vi "右相机穿管检测CCD2.vi"(8 "error in (no error)":errorcluster caption="错误输入（无错误）", 11 "名称或相对路径":string="Template Program") -> (0 "error in (no error) 2":errorcluster caption="错误输入（无错误）")   [LabVIEW 2017]
uses:
  Picture/SaveButtom.ctl
  <vilib>/vision/Pattern Matching.llb/IMAQ Curve Parameters.ctl
  Global System.vi
  <vilib>/Utility/xml.llb/Write to XML File(string).vi
panel:
  in  "ROI BIG 获取":bool
  in  "获取图像":bool
  in  "ROI LINE 获取":bool
  in  "创建模板":bool
  in  "保存图像":bool
  out "添加的路径":path
  in  "刷新":bool
  in  "测试按钮":bool
  in  "保存按钮":bool
  in  "Main":enum32{"主参数", "模板匹配参数 ", "CCD2 ROI参数", "测试效果"}(tab)
  in  "CCD2基础参数":T1={"IsNorImage"=TRUE, "Exposure Values"=100289, "ImagePath"=path "C:/Users/hedongpo/Desktop/514-hdp/Alignment Assemble System/Test Picture/B/3.bmp"} caption="参数界面" {"Exposure Values" scale=0.0..200000.0}
  in  "CCD2参数":T4={"Rectangle"={"Left"=1952, "Top"=146, "Right"=370, "Bottom"=2690, "Rotation"=45.0}, "Angle (degrees) "=90.0, "long"=150.0, "abgek"=-90.0, "Color"=16711680, "left threshold"=0.0, "Rectangle right"={"Left"=1952, "Top"=1596, "Right"=570, "Bottom"=2690, "Rotation"=45.0}, "long right"=150.0, "abgek right"=90.0, "Color 2"=16711680, "right threshold"=0.0, "left"=0.0, "right"=0.0, "Settings (Big)"={"Extraction Mode"=0, "Edge Threshold"=17, "Edge Filter Size"=1, "Min Length"=36, "Row Search Step Size"=13, "Col Search Step Size"=13, "Max Endpoint Gap"=10, "Closed"=FALSE, "Subpixel"=TRUE}, "Clamp Settings (Big)"={"Angle "=10.0, "Edge Polarity"={"Start"=0, "End"=0}}, " Settings top"={"Extraction Mode"=0, "Edge Threshold"=18, "Edge Filter Size"=1, "Min Length"=36, "Row Search Step Size"=64, "Col Search Step Size"=64, "Max Endpoint Gap"=10, "Closed"=FALSE, "Subpixel"=TRUE}, "Clamp Settings top "={"Angle "=10.0, "Edge Polarity"={"Start"=0, "End"=0}}, "Sub-Pixel Accuracy "=TRUE, "Threshold Parameters"={"Level Type"=enum."Absolute Value", "Threshold Level"=127, "Hysteresis"=2}, "Process "=enum."Get First + Last Edge", "Threshold Parameters 2"={"Level Type"=enum."Absolute Value", "Threshold Level"=127, "Hysteresis"=2}} {"Clamp Settings top"."Edge Polarity"."Start" items=["Any", "Rising", "Falling"]; "Clamp Settings top"."Edge Polarity"."End" items=["Any", "Rising", "Falling"]; "Settings top"."Extraction Mode" items=["Normal", "Uniform Regions"]; "Settings top"."Edge Filter Size" items=["Fine", "Normal", "Contour Tracing"]; "Settings top"."Max Endpoint Gap" min=0; "Settings top"."Col Search Step Size" min=1 max=255 step=1; "Settings top"."Row Search Step Size" min=1 max=255 step=1; "Settings top"."Min Length" min=0; "Settings top"."Edge Threshold" min=1 max=350 step=1; "Clamp Settings (Big)"."Edge Polarity"."Start" items=["Any", "Rising", "Falling"]; "Clamp Settings (Big)"."Edge Polarity"."End" items=["Any", "Rising", "Falling"]; "Settings (Big)"."Extraction Mode" items=["Normal", "Uniform Regions"]; "Settings (Big)"."Edge Filter Size" items=["Fine", "Normal", "Contour Tracing"]; "Settings (Big)"."Max Endpoint Gap" min=0; "Settings (Big)"."Col Search Step Size" min=1 max=255 step=1; "Settings (Big)"."Row Search Step Size" min=1 max=255 step=1; "Settings (Big)"."Min Length" min=0; "Settings (Big)"."Edge Threshold" min=1 max=350 step=1; "Rectangle right"."Rotation" format="%.2f"; "Rectangle right"."Left" scale=0.0..1024.0; "Rectangle right"."Right" scale=0.0..1024.0; "Rectangle"."Rotation" format="%.2f"; "Rectangle"."Left" scale=0.0..1024.0; "Rectangle"."Right" scale=0.0..1024.0}
  in  "CCD2 ROI参数":T6={"Rectangle big CCD1"={"Left"=1952, "Top"=1596, "Right"=570, "Bottom"=2690, "Rotation"=45.0}, "Rectangle top CCD1 "={"Left"=1952, "Top"=1596, "Right"=570, "Bottom"=2690, "Rotation"=45.0}, "Line"={"Start X"=0, "Start Y"=0, "End X"=0, "End Y"=0}, "left line "=846.0, "right line"=1152.0} {"Line"."Start X" scale=0.0..1024.0; "Line"."End X" scale=0.0..1024.0; "Rectangle top CCD1"."Rotation" format="%.2f"; "Rectangle top CCD1"."Left" scale=0.0..1024.0; "Rectangle top CCD1"."Right" scale=0.0..1024.0; "Rectangle big CCD1"."Rotation" format="%.2f"; "Rectangle big CCD1"."Left" scale=0.0..1024.0; "Rectangle big CCD1"."Right" scale=0.0..1024.0}
  out "原始图像":T7(plugin-control)
  out "路径输出":path
  in  "Vision Paramter Save Buttom":T8
  out "system time":string
  in  "确认按钮":bool
  # "箭头指示参数"
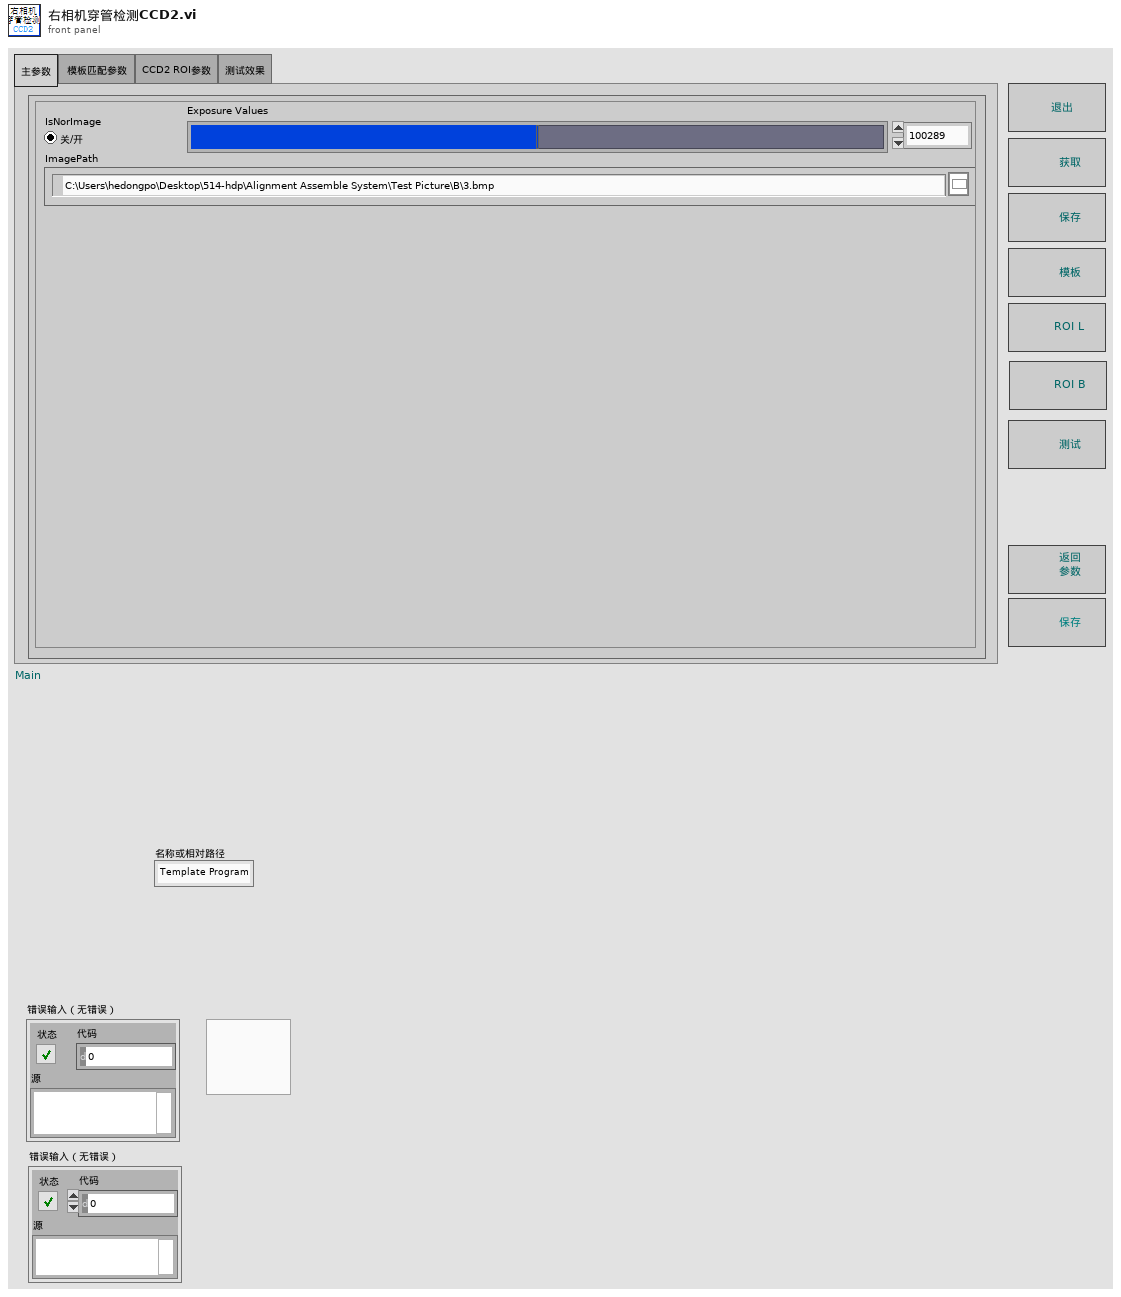
[diagram p1: front panel]
types:
  T1 = cluster{"IsNorImage":bool, "Exposure Values":u32, "ImagePath":path}
  T2 = typedef "IMAQ Rectangle" = cluster{"Left":i32, "Top":i32, "Right":i32, "Bottom":i32, "Rotation":dbl}
  T3 = typedef "IMAQ Curve Parameters.ctl" = cluster{"Extraction Mode":u32, "Edge Threshold":i32, "Edge Filter Size":u32, "Min Length":i32, "Row Search Step Size":i32, "Col Search Step Size":i32, "Max Endpoint Gap":i32, "Closed":bool, "Subpixel":bool}
  T4 = cluster{"Rectangle":T2, "Angle (degrees) ":sgl, "long":sgl, "abgek":dbl, "Color":u32, "left threshold":dbl, "Rectangle right":T2, "long right":sgl, "abgek right":dbl, "Color 2":u32, "right threshold":dbl, "left":dbl, "right":dbl, "Settings (Big)":T3, "Clamp Settings (Big)":cluster{"Angle ":dbl, "Edge Polarity":cluster{"Start":u32, "End":u32}}, " Settings top":T3, "Clamp Settings top ":cluster{"Angle ":dbl, "Edge Polarity":cluster{"Start":u32, "End":u32}}, "Sub-Pixel Accuracy ":bool, "Threshold Parameters":cluster{"Level Type":enum32{"Absolute Value", "Relative value"}, "Threshold Level":i32, "Hysteresis":i32}, "Process ":enum16{"Get First Edge", "Get First + Last Edge", "Get All Edges"}, "Threshold Parameters 2":cluster{"Level Type":enum32{"Absolute Value", "Relative value"}, "Threshold Level":i32, "Hysteresis":i32}}
  T5 = typedef "IMAQ Line" = cluster{"Start X":i32, "Start Y":i32, "End X":i32, "End Y":i32}
  T6 = cluster{"Rectangle big CCD1":T2, "Rectangle top CCD1 ":T2, "Line":T5, "left line ":dbl, "right line":dbl}
  T7 = typedef "IMAQ Image.ctl" = refnum<image>
  T8 = typedef "SaveButtom.ctl" = bool
  T9 = cluster{"index":i32, "this vi":refnum<vi>, "error out":errorcluster}
  T10 = cluster{"master data":string, "priority":u16, "secondary data":string[]}
  T11 = cluster{"case name":string[], "queue array":refnum<queue>[]}
  T12 = typedef "IMAQdx.ctl" = refnum<k21>
  T13 = cluster{"Global Rectangle":i32[], "Contours":cluster{"Contour Type":u32, "ROI Type":u32, "Points":i32[]}[]}
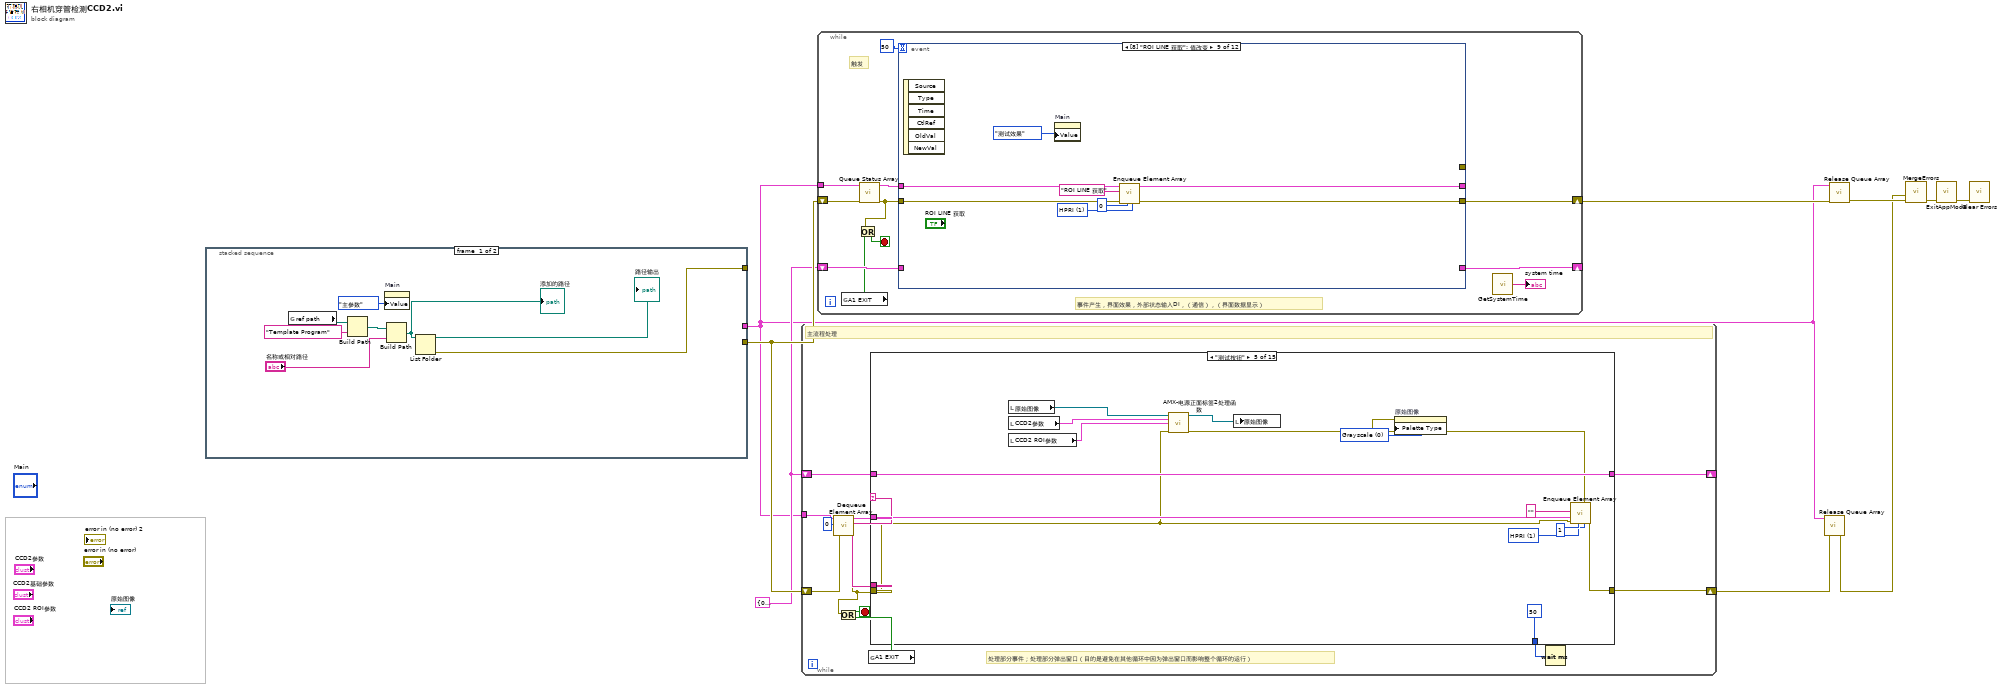
[diagram p0: block diagram]
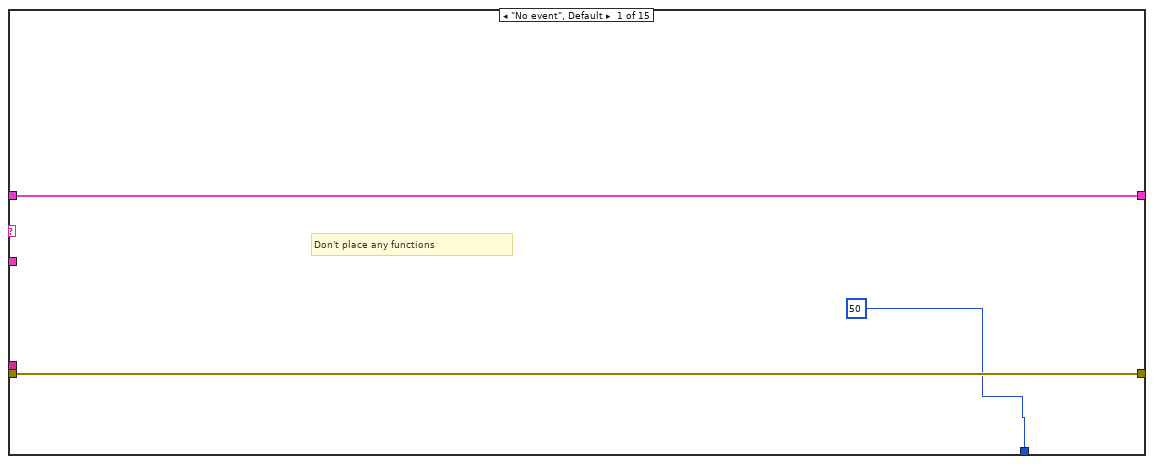
[diagram p2: hidden frame]
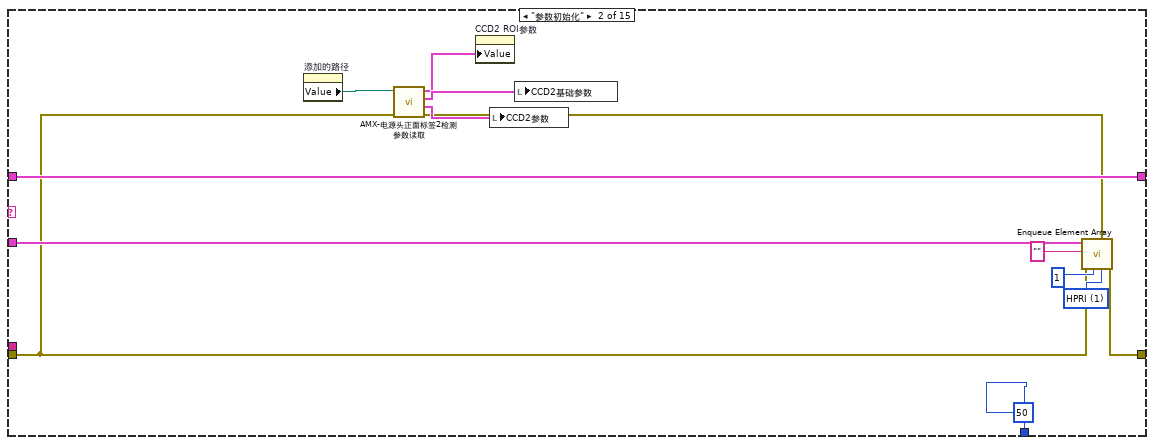
[diagram p3: hidden frame]
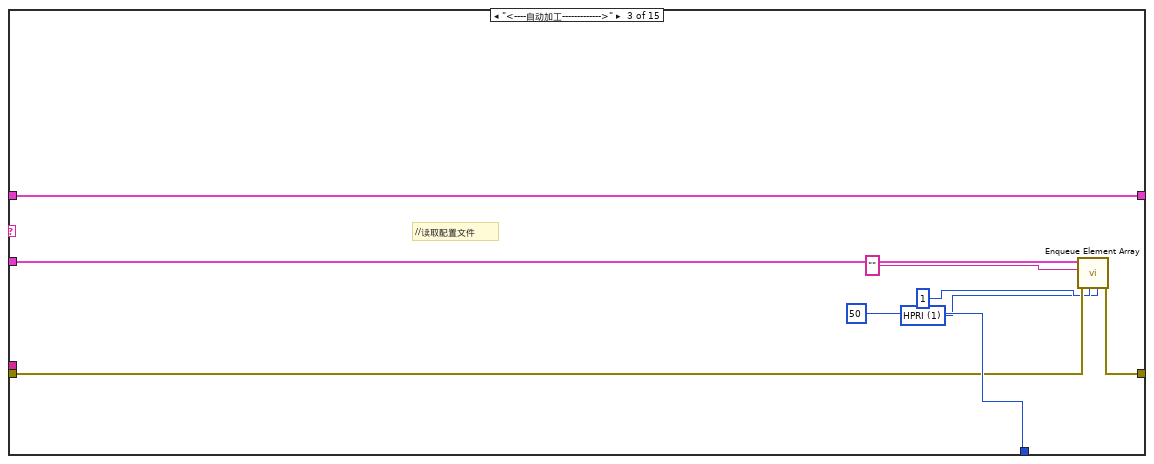
[diagram p4: hidden frame]
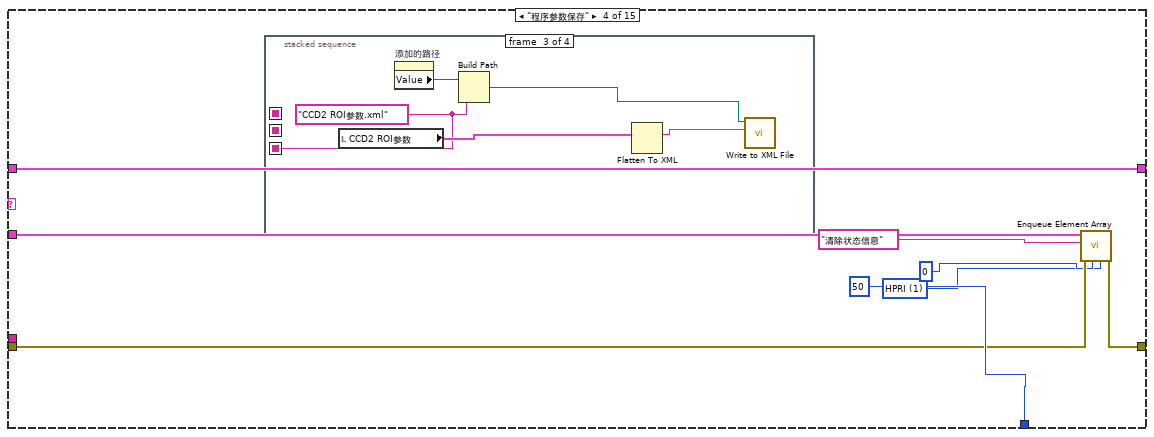
[diagram p5: hidden frame]
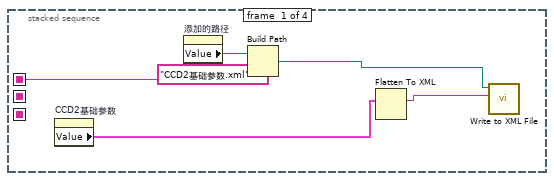
[diagram p6: hidden frame]
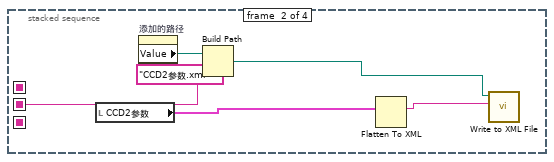
[diagram p7: hidden frame]
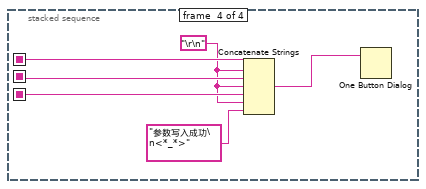
[diagram p8: hidden frame]
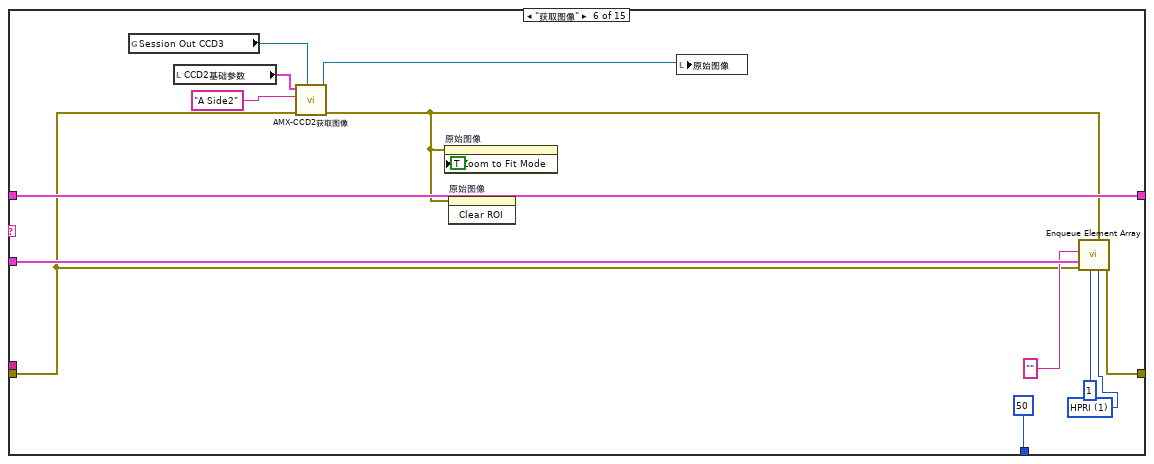
[diagram p9: hidden frame]
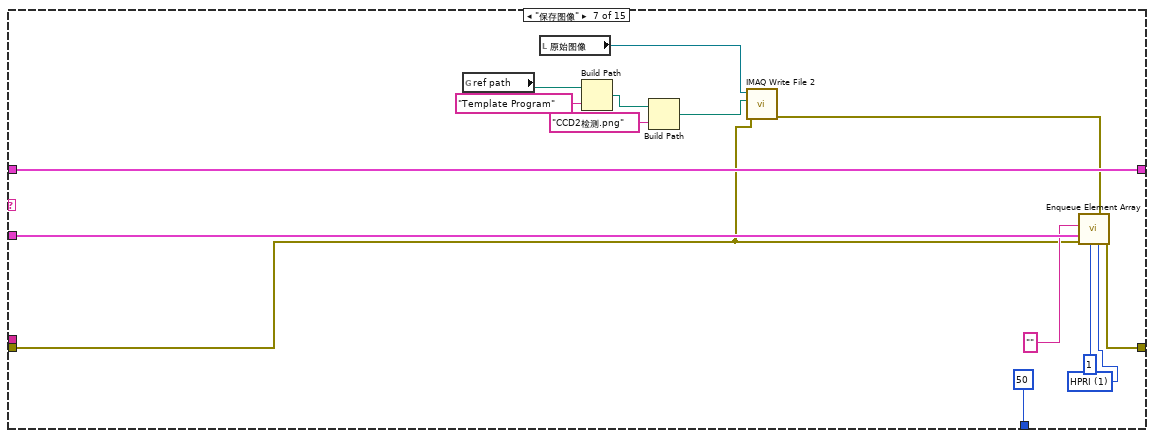
[diagram p10: hidden frame]
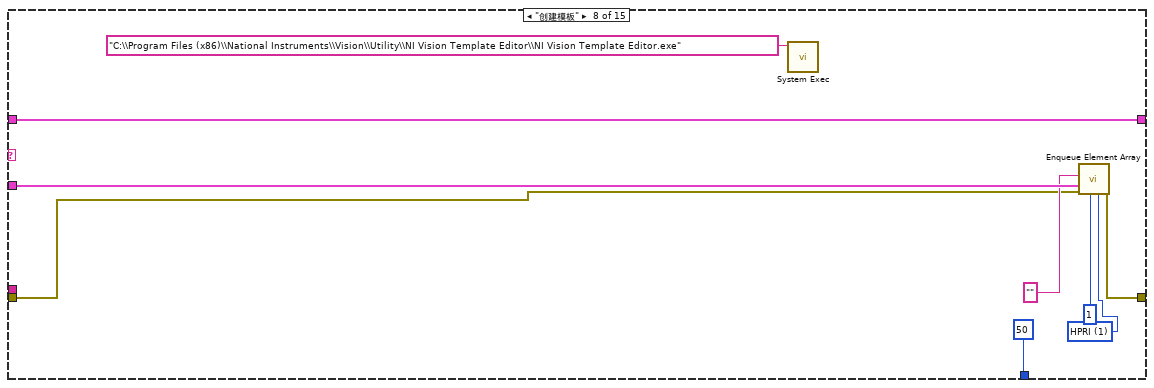
[diagram p11: hidden frame]
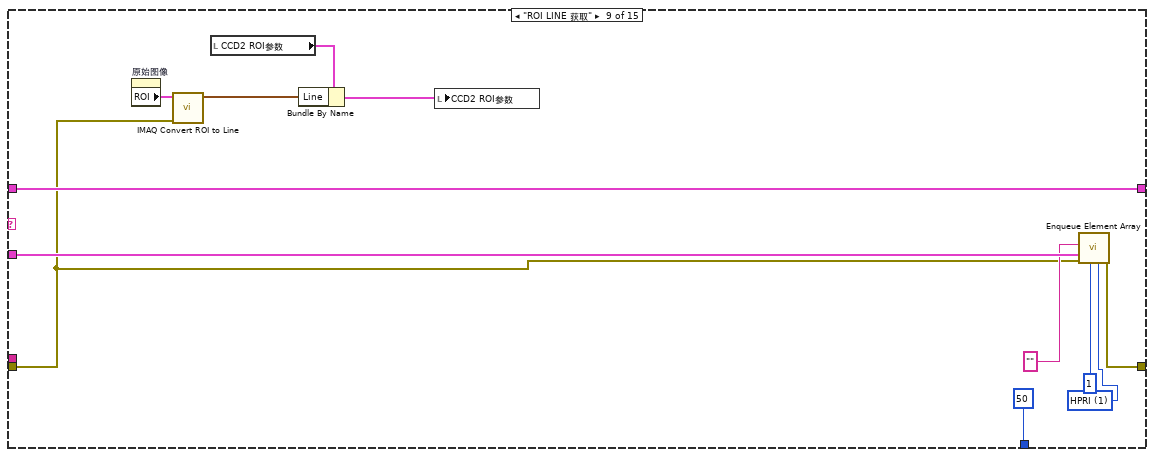
[diagram p12: hidden frame]
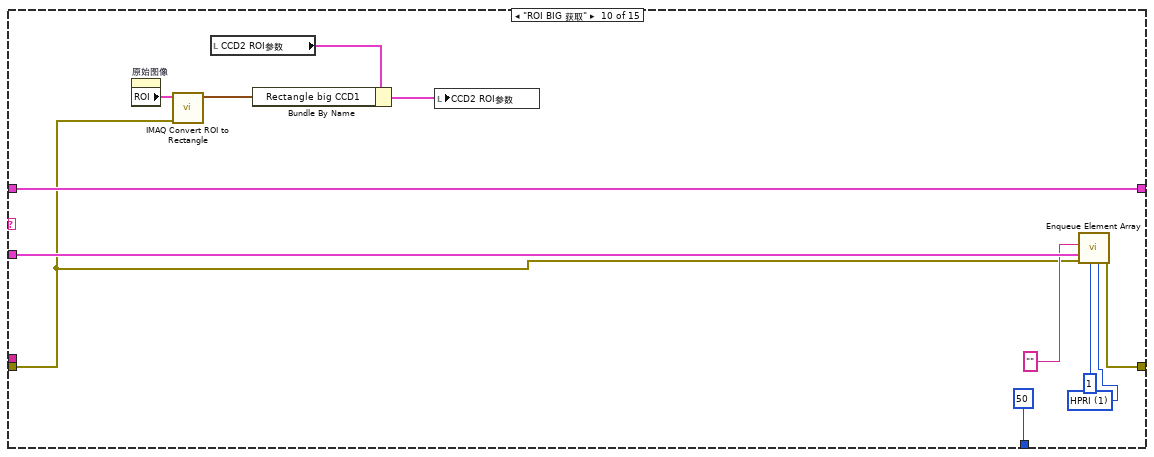
[diagram p13: hidden frame]
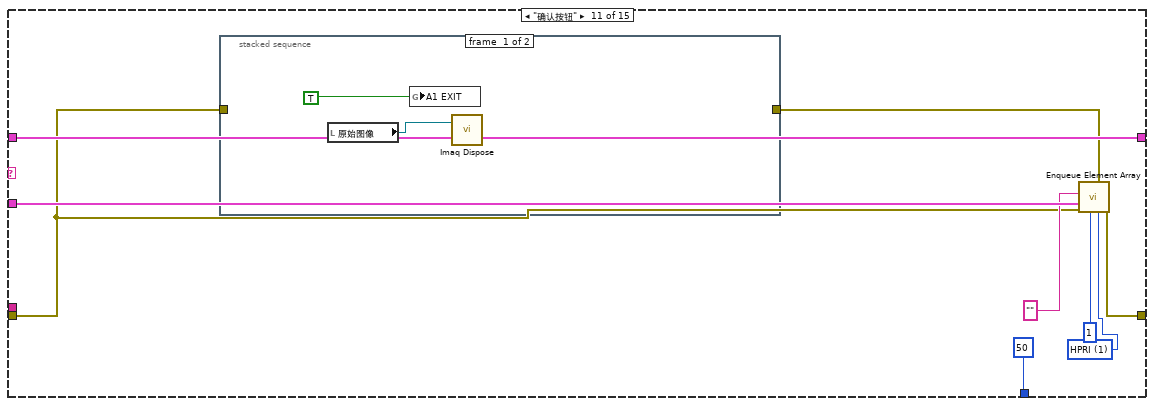
[diagram p14: hidden frame]
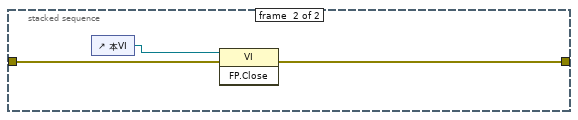
[diagram p15: hidden frame]
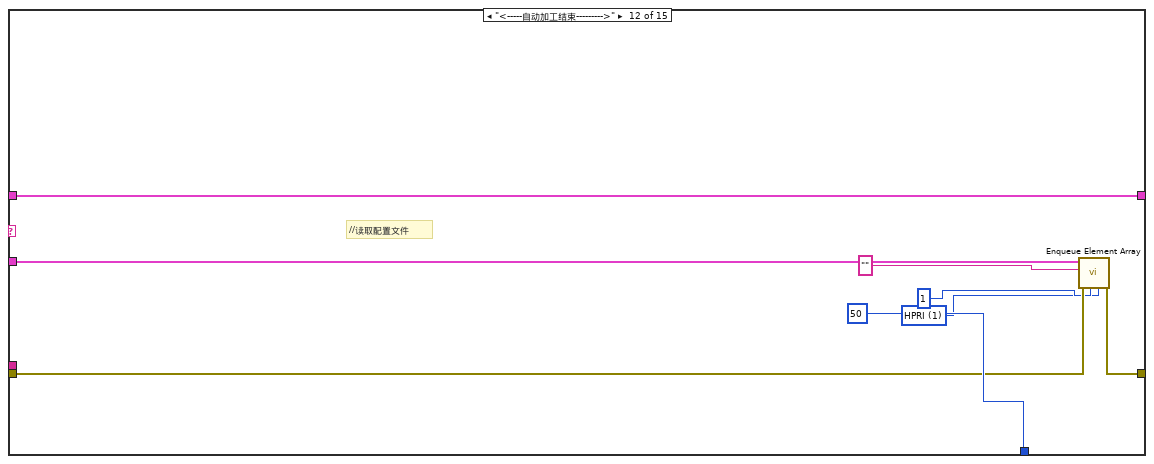
[diagram p16: hidden frame]
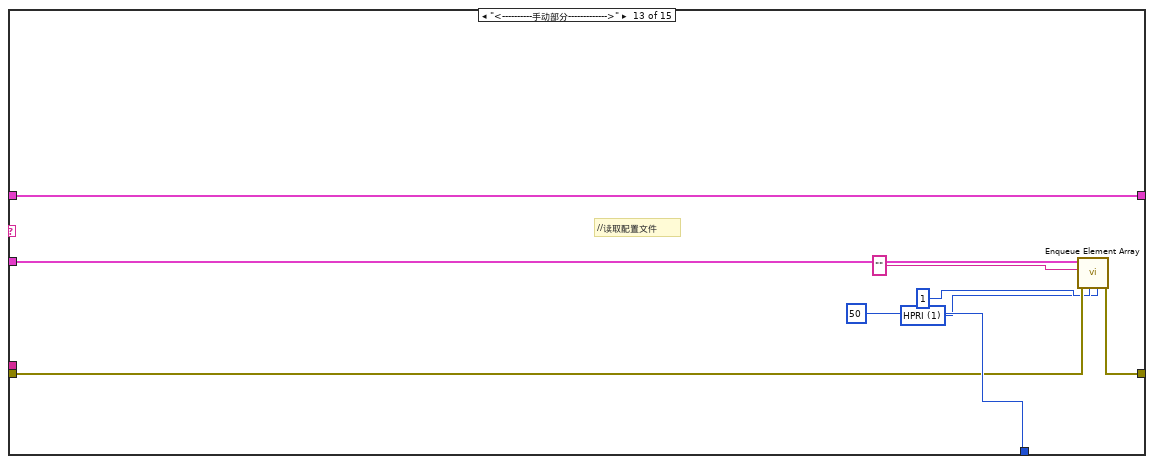
[diagram p17: hidden frame]
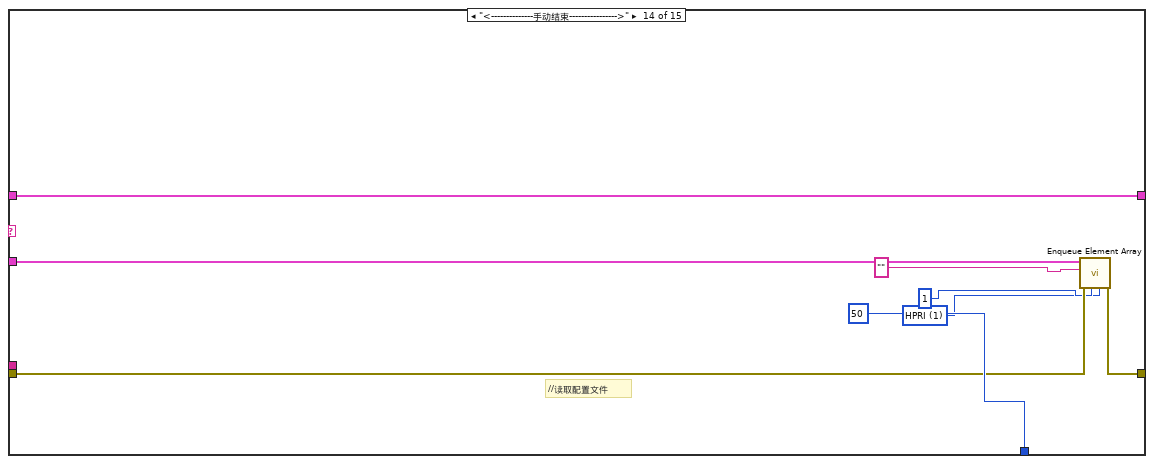
[diagram p18: hidden frame]
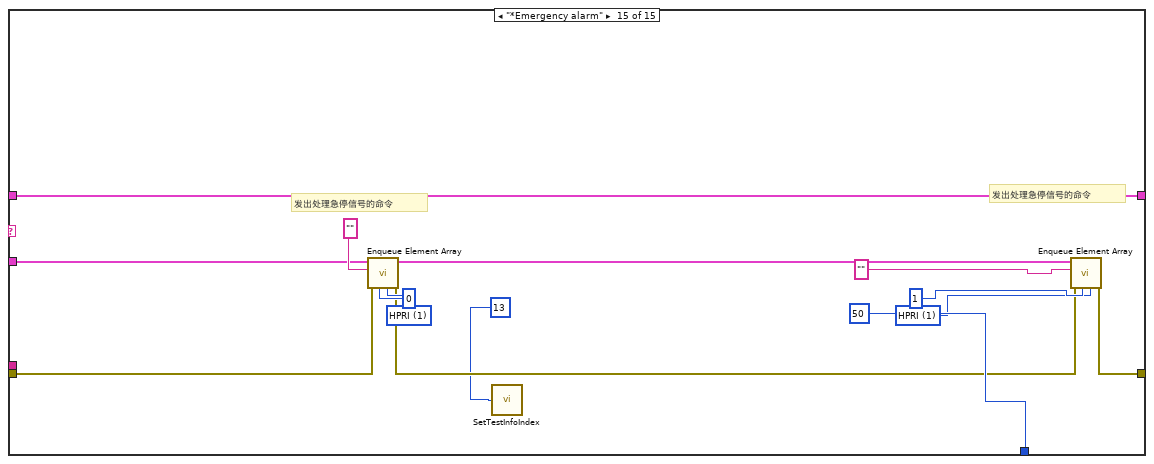
[diagram p19: hidden frame]
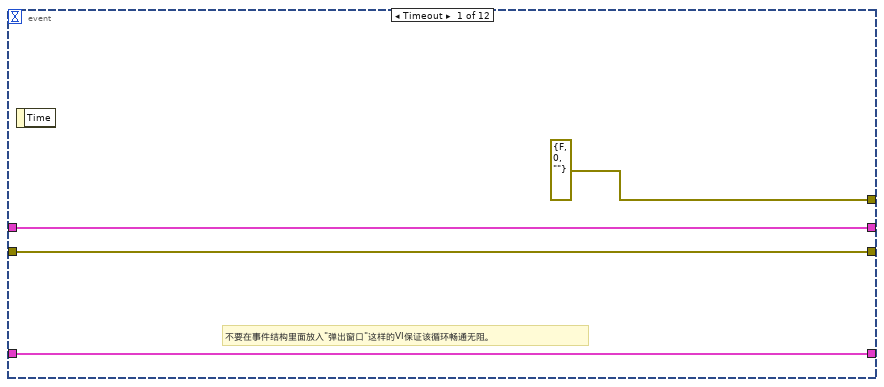
[diagram p20: hidden frame]
diagram:
  w4 = T9 {"index"=0, "this vi"=refnum, "error out"={"status"=FALSE, "code"=0, "source"=""}} ("parameter buffer")
  n1 = stacked-sequence {
    tunnel: [w15 _] -> _
    tunnel: [_ w19] -> w5
    tunnel: [_ w18] -> w1
    frame #0 {
      n2 = global read "Global System.vi" "ref path"() -> (w13:path)
      n3 = Build Path(base path=w13, name or relative path="Template Program" ("名称或相对路径")) -> (appended path=w11:path)
      n4 = property on="Main" class="TabCtl (严格)"("Value"=enum32{"主参数", "模板匹配参数 ", "CCD2 ROI参数", "测试效果"}."主参数" ("Main")) -> ()  [unwired: 2 in, 2 out]
      n5 = Build Path(base path=w11, name or relative path="名称或相对路径") -> (appended path=w17:path)
      "添加的路径" <- w17
      n6 = List Folder(path=w17) -> (path out=→"路径输出":path, error out=w15:errorcluster)  [unwired: 3 in, 2 out]
    }
    frame #1 {
      w27 = string[] ["comm queue1", "data queue 11", "data queue 12", "data queue 13", "data queue 14"]  # queue name
      w28 = 4  # queue num
      w29 = T10 {"master data"="", "priority"=0, "secondary data"=[]}  # element data type
      n7 = call "Obtain Queue Array.vi"("queue name"=w27, "element data type"=w29, "queue num"=w28) -> ("error out"=w23:errorcluster, "queue out"=w24:T11)  [unwired: 2 in, 1 out]
      n8 = call "Enqueue Element Array.vi"("queue index"=0, "error in"=w23, "master data"="参数初始化", "queue in"=w24) -> ("error out"=w22:errorcluster, "queue out"=w21:T11)  [unwired: 6 in]
      n9 = disable-structure shown="启用" {
        disable-tunnel: w22 -> [w35 w36]
        disable-tunnel: w21 -> [w34 w37]
        disable-tunnel: "Loading Variable" ("master data") -> [w33 _]
        disable-tunnel: [w31 w36] -> w19
        disable-tunnel: [w30 w37] -> w18
        frame Disabled {
          n10 = call "Enqueue Element Array.vi"("queue index"=12, "error in"=w35, "master data"=w33, "queue in"=w34) -> ("error out"=w31:errorcluster, "queue out"=w30:T11)  [unwired: 6 in]
        }
        frame Enabled {
        }
      }
    }
  }
  n11 = while {
    shift-right: [w50] -> w3
    shift-left: w5 -> [w41]
    shift-right: [w47] -> _
    shift-left: w4 -> [w48]
    tunnel: w1 -> [w43]
    stop <- w38 stop-if-true
    # "处理部分事件；处理部分弹出窗口（目的是避免在其他循环中因为弹出窗口而影响整个循环的运行）"
    # "主流程处理"
    n12 = call "Dequeue Element Array.vi"("queue in"=w43, "queue index"=0, "error in"=w41) -> ("queue out"=w46:T11, "master data"=w45:string, "secondary data"=w44:string[], "error out"=w40:errorcluster)  [unwired: 2 in, 1 out]
    n13 = global read "Global System.vi" "A1 EXIT"() -> (w39:bool)
    n14 = Or(x=w40, y=w39) -> (x .or. y?=w38:bool)
    n15 = case shown="\"测试按钮\"" w45 {
      tunnel: w46 -> [_ w65 w73 w75 w116 w130 w145 w154 w166 w178 w187 w200 w208 w216 w222]
      tunnel: w40 -> [w52 w58 w69 w79 w110 w121 w132 w148 w159 w171 w181 w196 w204 w212 w219]
      tunnel: [w52 w64 w72 w81 w115 w129 w144 w153 w165 w177 w186 w199 w207 w215 w230] -> w50
      tunnel: [50 50 50 50 50 50 50 50 50 50 50 50 50 50 50] -> w49
      tunnel: w48 -> [w53 w60 w70 w76 w111 w125 w140 w149 w161 w173 w182 w197 w205 w213 w228]
      tunnel: [w53 w60 w70 w76 w111 w125 w140 w149 w161 w173 w182 w197 w205 w213 w228] -> w47
      tunnel: w44 -> [_ _ _ _ _ _ _ _ _ _ _ _ _ _ _]
      frame "No event", Default {
        # "Don't place any functions"
      }
      frame "参数初始化" {
        w61 = u16 1 items=["HPRI"=1, "LPRI"=0] ("priority")
        n16 = property on="添加的路径" class="Path"() -> ("Value"=w59:path)  [unwired: 2 in, 2 out]
        n17 = call "AMX-电源头正面标签2检测参数读取.vi"("error in (no error)"=w58, "基路径"=w59) -> ("error out"=w55:errorcluster, "CCD2参数"=w56:T4, "CCD2基础参数"=w57:T1, "CCD2 ROI参数"=w54:T6)  [unwired: 5 in]
        n18 = property on="CCD2 ROI参数" class="Clust (严格)"("Value"=w54) -> ()  [unwired: 2 in, 2 out]
        n19 = local write "CCD2参数"(w56) -> ()
        n20 = local write "CCD2基础参数"(w57) -> ()
        n21 = call "Enqueue Element Array.vi"("priority"=w61, "device error in"=w55, "queue index"=1, "error in"=w58, "master data"="" ("Element 1"), "queue in"=w65) -> ("error out"=w64:errorcluster)  [unwired: 4 in, 1 out]
      }
      frame "<----自动加工------------->" {
        w67 = u16 1 items=["HPRI"=1, "LPRI"=0] ("priority")
        # "//读取配置文件"
        n22 = call "Enqueue Element Array.vi"("priority"=w67, "queue index"=1, "error in"=w69, "master data"="" ("Element 1"), "queue in"=w73) -> ("error out"=w72:errorcluster)  [unwired: 5 in, 1 out]
      }
      frame "程序参数保存" {
        w77 = u16 1 items=["HPRI"=1, "LPRI"=0] ("priority")
        n23 = stacked-sequence {
          seq-local: [w83 _ _ _] -> [_ _ _ w103]
          seq-local: [_ w89 _ _] -> [_ _ _ w101]
          seq-local: [_ _ w93 _] -> [_ _ _ w99]
          frame #0 {
            w83 = "CCD2基础参数.xml" ("名称或相对路径")
            n24 = property on="CCD2基础参数" class="Clust (严格)"() -> ("Value"=w86:T1)  [unwired: 2 in, 2 out]
            n25 = property on="添加的路径" class="Path"() -> ("Value"=w87:path)  [unwired: 2 in, 2 out]
            n26 = Build Path(base path=w87, name or relative path=w83) -> (appended path=w84:path)
            n27 = Flatten To XML(anything=w86) -> (xml string=w85:string)
            n28 = call-poly <vilib>:"Write to XML File.vi"("XML Input"=w85, "XML File Path"=w84) -> ()  [unwired: 7 in, 3 out]
          }
          frame #1 {
            w89 = "CCD2参数.xml" ("名称或相对路径")
            n29 = local read "CCD2参数"() -> (w88:T4)
            n30 = property on="添加的路径" class="Path"() -> ("Value"=w92:path)  [unwired: 2 in, 2 out]
            n31 = Build Path(base path=w92, name or relative path=w89) -> (appended path=w90:path)
            n32 = Flatten To XML(anything=w88) -> (xml string=w91:string)
            n33 = call-poly <vilib>:"Write to XML File.vi"("XML Input"=w91, "XML File Path"=w90) -> ()  [unwired: 7 in, 3 out]
          }
          frame #2 {
            w93 = "CCD2 ROI参数.xml" ("名称或相对路径")
            n34 = local read "CCD2 ROI参数"() -> (w94:T6)
            n35 = property on="添加的路径" class="Path"() -> ("Value"=w97:path)  [unwired: 2 in, 2 out]
            n36 = Build Path(base path=w97, name or relative path=w93) -> (appended path=w95:path)
            n37 = Flatten To XML(anything=w94) -> (xml string=w96:string)
            n38 = call-poly <vilib>:"Write to XML File.vi"("XML Input"=w96, "XML File Path"=w95) -> ()  [unwired: 7 in, 3 out]
          }
          frame #3 {
            w98 = "\r\n"
            n39 = Concatenate Strings(w103, w98, w101, w98, w99, w98, "参数写入成功\n<*_*>" ("消息")) -> (w102:string)
            n40 = One Button Dialog(message=w102) -> ()  [unwired: 1 in, 1 out]
          }
        }
        n41 = call "Enqueue Element Array.vi"("priority"=w77, "queue index"=0, "error in"=w79, "master data"="清除状态信息" ("Element 1"), "queue in"=w75) -> ("error out"=w81:errorcluster)  [unwired: 5 in, 1 out]
      }
      frame "测试按钮" {
        w106 = u32 0 items=["Grayscale", "Binary", "Gradient", "Rainbow", "Temperature", "User Defined", "Binary 16 Bit", "Gradient 16 Bit", "Rainbow 16 Bit", "Temperature 16 Bit", "User Defined 16 Bit"] ("Palette:Palette Type")
        w112 = u16 1 items=["HPRI"=1, "LPRI"=0] ("priority")
        n42 = local read "原始图像"() -> (w108:T7)
        n43 = local read "CCD2参数"() -> (w105:T4)
        n44 = local read "CCD2 ROI参数"() -> (w104:T6)
        n45 = call "AMX-电源正面标签2处理函数.vi"("Image in"=w108, "CCD2参数"=w105, "CCD2 ROI参数"=w104, "error in (no error)"=w110) -> ("Image out"=w109:T7, "error out"=w107:errorcluster)  [unwired: 7 in, 3 out]
        n46 = local write "原始图像"(w109) -> ()
        n47 = property on="原始图像" class="ImageControl"(error in=w107, "Palette Type"=w106) -> ()  [unwired: 1 in, 2 out]
        n48 = call "Enqueue Element Array.vi"("priority"=w112, "device error in"=w107, "queue index"=1, "error in"=w110, "master data"="" ("Element 1"), "queue in"=w116) -> ("error out"=w115:errorcluster)  [unwired: 4 in, 1 out]
      }
      frame "获取图像" {
        w126 = u16 1 items=["HPRI"=1, "LPRI"=0] ("priority")
        n49 = global read "Global System.vi" "Session Out CCD3"() -> (w118:T12)
        n50 = local read "CCD2基础参数"() -> (w123:T1)
        n51 = call "AMX-CCD2获取图像.vi"("Session Out CCD3"=w118, "error in (no error)"=w121, "Image Name"="A Side2", "ParamsUI"=w123) -> ("error out"=w119:errorcluster, "Image out"=w122:T7)  [unwired: 4 in, 2 out]
        n52 = property on="原始图像" class="ImageControl"(error in=w119, "Zoom to Fit Mode"=TRUE) -> ()  [unwired: 1 in, 2 out]
        n53 = invoke on="原始图像" class="ImageControl" method="Clear ROI"(error in=w119) -> ()  [unwired: 2 in, 3 out]
        n54 = local write "原始图像"(w122) -> ()
        n55 = call "Enqueue Element Array.vi"("priority"=w126, "device error in"=w119, "queue index"=1, "error in"=w121, "master data"="" ("Element 1"), "queue in"=w130) -> ("error out"=w129:errorcluster)  [unwired: 4 in, 1 out]
      }
      frame "保存图像" {
        w141 = u16 1 items=["HPRI"=1, "LPRI"=0] ("priority")
        n56 = global read "Global System.vi" "ref path"() -> (w139:path)
        n57 = local read "原始图像"() -> (w133:T7)
        n58 = Build Path(base path=w139, name or relative path="Template Program" ("名称或相对路径")) -> (appended path=w137:path)
        n59 = Build Path(base path=w137, name or relative path="CCD2检测.png" ("名称或相对路径")) -> (appended path=w135:path)
        n60 = call-poly "IMAQ Write File 2"("error in (no error)"=w132, "File Path"=w135, "Image"=w133) -> ("error out"=w134:errorcluster)  [unwired: 7 in, 1 out]
        n61 = call "Enqueue Element Array.vi"("priority"=w141, "device error in"=w134, "queue index"=1, "error in"=w132, "master data"="" ("Element 1"), "queue in"=w145) -> ("error out"=w144:errorcluster)  [unwired: 4 in, 1 out]
      }
      frame "创建模板" {
        w150 = u16 1 items=["HPRI"=1, "LPRI"=0] ("priority")
        n62 = call <vilib>:"System Exec.vi"("command line"="C:\\Program Files (x86)\\National Instruments\\Vision\\Utility\\NI Vision Template Editor\\NI Vision Template Editor.exe") -> ()  [unwired: 7 in, 4 out]
        n63 = call "Enqueue Element Array.vi"("priority"=w150, "queue index"=1, "error in"=w148, "master data"="" ("Element 1"), "queue in"=w154) -> ("error out"=w153:errorcluster)  [unwired: 5 in, 1 out]
      }
      frame "ROI LINE 获取" {
        w162 = u16 1 items=["HPRI"=1, "LPRI"=0] ("priority")
        n64 = property on="原始图像" class="ImageControl"() -> ("ROI"=w160:T13)  [unwired: 2 in, 2 out]
        n65 = call "IMAQ Convert ROI to Line"("error in (no error)"=w159, "ROI Descriptor"=w160) -> ("Line"=w157:T5)  [unwired: 7 in, 1 out]
        n66 = local read "CCD2 ROI参数"() -> (w158:T6)
        n67 = Bundle By Name(cluster=w158, "Line"=w157) -> (w156:T6)
        n68 = local write "CCD2 ROI参数"(w156) -> ()
        n69 = call "Enqueue Element Array.vi"("priority"=w162, "queue index"=1, "error in"=w159, "master data"="" ("Element 1"), "queue in"=w166) -> ("error out"=w165:errorcluster)  [unwired: 5 in, 1 out]
      }
      frame "ROI BIG 获取" {
        w174 = u16 1 items=["HPRI"=1, "LPRI"=0] ("priority")
        n70 = property on="原始图像" class="ImageControl"() -> ("ROI"=w172:T13)  [unwired: 2 in, 2 out]
        n71 = call "IMAQ Convert ROI to Rectangle"("error in (no error)"=w171, "ROI Descriptor"=w172) -> ("Rectangle"=w169:T2)  [unwired: 7 in, 1 out]
        n72 = local read "CCD2 ROI参数"() -> (w170:T6)
        n73 = Bundle By Name(cluster=w170, "Rectangle big CCD1"=w169) -> (w168:T6)
        n74 = local write "CCD2 ROI参数"(w168) -> ()
        n75 = call "Enqueue Element Array.vi"("priority"=w174, "queue index"=1, "error in"=w171, "master data"="" ("Element 1"), "queue in"=w178) -> ("error out"=w177:errorcluster)  [unwired: 5 in, 1 out]
      }
      frame "确认按钮" {
        w183 = u16 1 items=["HPRI"=1, "LPRI"=0] ("priority")
        n76 = stacked-sequence {
          tunnel: w181 -> [_ w192]
          tunnel: [_ w191] -> w180
          frame #0 {
            n77 = local read "原始图像"() -> (w189:T7)
            n78 = global write "Global System.vi" "A1 EXIT"(TRUE ("EXIT")) -> ()
            n79 = call "Imaq Dispose"("Image"=w189) -> ()  [unwired: 5 in, 1 out]
          }
          frame #1 {
            n80 = control-ref of="本VI"() -> (w193:refnum<vi>)
            n81 = invoke class="VI" method="FP.Close"(reference=w193, error in=w192) -> (error out=w191:errorcluster)  [unwired: 1 in, 2 out]
          }
        }
        n82 = call "Enqueue Element Array.vi"("priority"=w183, "device error in"=w180, "queue index"=1, "error in"=w181, "master data"="" ("Element 1"), "queue in"=w187) -> ("error out"=w186:errorcluster)  [unwired: 4 in, 1 out]
      }
      frame "<-----自动加工结束--------->" {
        w194 = u16 1 items=["HPRI"=1, "LPRI"=0] ("priority")
        # "//读取配置文件"
        n83 = call "Enqueue Element Array.vi"("priority"=w194, "queue index"=1, "error in"=w196, "master data"="" ("Element 1"), "queue in"=w200) -> ("error out"=w199:errorcluster)  [unwired: 5 in, 1 out]
      }
      frame "<----------手动部分------------->" {
        w202 = u16 1 items=["HPRI"=1, "LPRI"=0] ("priority")
        # "//读取配置文件"
        n84 = call "Enqueue Element Array.vi"("priority"=w202, "queue index"=1, "error in"=w204, "master data"="" ("Element 1"), "queue in"=w208) -> ("error out"=w207:errorcluster)  [unwired: 5 in, 1 out]
      }
      frame "<--------------手动结束---------------->" {
        w210 = u16 1 items=["HPRI"=1, "LPRI"=0] ("priority")
        # "//读取配置文件"
        n85 = call "Enqueue Element Array.vi"("priority"=w210, "queue index"=1, "error in"=w212, "master data"="" ("Element 1"), "queue in"=w216) -> ("error out"=w215:errorcluster)  [unwired: 5 in, 1 out]
      }
      frame "*Emergency alarm" {
        w225 = u16 1 items=["HPRI"=1, "LPRI"=0] ("priority")
        w226 = u16 1 items=["HPRI"=1, "LPRI"=0] ("priority")
        # "发出处理急停信号的命令"
        # "发出处理急停信号的命令"
        n86 = call "Enqueue Element Array.vi"("priority"=w225, "queue index"=0, "error in"=w219, "master data"="" ("Element 1"), "queue in"=w222) -> ("error out"=w220:errorcluster, "queue out"=w221:T11)  [unwired: 5 in]
        n87 = call "SetTestInfoIndex.vi"("test info index"=13) -> ()
        n88 = call "Enqueue Element Array.vi"("priority"=w226, "queue index"=1, "error in"=w220, "master data"="" ("Element 1"), "queue in"=w221) -> ("error out"=w230:errorcluster)  [unwired: 5 in, 1 out]
      }
    }
    n89 = Wait (ms)(milliseconds to wait=w49) -> ()  [unwired: 1 out]
  }
  n90 = while {
    shift-right: [w235] -> w6
    shift-left: w5 -> [w239]
    shift-right: [w237] -> _
    shift-left: w4 -> [w238]
    tunnel: w1 -> [w241]
    stop <- w232 stop-if-true
    # "触发"
    # "事件产生，界面效果，外部状态输入DI，（通信），（界面数据显示）"
    n91 = global read "Global System.vi" "A1 EXIT"() -> (w233:bool)
    n92 = call "Queue Status Array.vi"("error in (no error)"=w239, "queue in"=w241) -> ("error out"=w234:errorcluster, "queue out"=w236:T11)  [unwired: 4 in]
    n93 = Or(x=w234, y=w233) -> (x .or. y?=w232:bool)
    n94 = event shown="[8] \"ROI LINE 获取\": 值改变" {
      selector: _ -> [_ _ _ _ _ _ _ _ _ _ _ _]
      dyn-events: _ -> [_ _ _ _ _ _ _ _ _ _ _ _]
      timeout: 50 -> [_ _ _ _ _ _ _ _ _ _ _ _]
      tunnel: w238 -> [w246 w254 _ _ _ _ _ _ _ _ _ _]
      tunnel: [w246 w254 _ _ _ _ _ _ _ _ _ _] -> w237
      tunnel: [errorcluster {"status"=FALSE, "code"=0, "source"=""} ("error out") _ _ _ _ _ _ _ _ _ _ _] -> _
      tunnel: w236 -> [w244 w253 w259 w266 w273 w281 w288 w295 w303 w311 w319 w330]
      tunnel: w234 -> [w243 w252 w258 w265 w272 w280 w287 w294 w302 w310 w318 w329]
      tunnel: [w243 w251 w256 w263 w270 w278 w285 w292 w300 w308 w316 w327] -> w235
      tunnel: [w244 w250 w257 w264 w271 w279 w286 w293 w301 w309 w317 w328] -> _
      event Timeout {
        # "不要在事件结构里面放入\"弹出窗口\"这样的VI保证该循环畅通无阻。"
        n95 = event-data() -> ()  [unwired: 1 in, 1 out]
      }
      event Panel Close? {
        w248 = u16 1 items=["HPRI"=1, "LPRI"=0] ("priority")
        n96 = event-data() -> ()  [unwired: 1 in, 4 out]
        n97 = call "Enqueue Element Array.vi"("priority"=w248, "queue index"=0, "error in"=w252, "master data"="*Exit application", "queue in"=w253) -> ("error out"=w251:errorcluster, "queue out"=w250:T11)  [unwired: 5 in]
        n98 = event-data("Discard?"=TRUE) -> ()  [unwired: 1 in, 1 out]
      }
      event Value Change {
        w261 = u16 1 items=["HPRI"=1, "LPRI"=0] ("priority")
        n99 = event-data() -> ()  [unwired: 1 in, 6 out]
        n100 = call "Enqueue Element Array.vi"("priority"=w261, "queue index"=0, "error in"=w258, "master data"="Vision Paramter Save", "queue in"=w259) -> ("error out"=w256:errorcluster, "queue out"=w257:T11)  [unwired: 5 in]
      }
      event "确认按钮": Value Change {
        w268 = u16 1 items=["HPRI"=1, "LPRI"=0] ("priority")
        n101 = event-data() -> ()  [unwired: 1 in, 6 out]
        n102 = call "Enqueue Element Array.vi"("priority"=w268, "queue index"=0, "error in"=w265, "master data"="确认按钮", "queue in"=w266) -> ("error out"=w263:errorcluster, "queue out"=w264:T11)  [unwired: 5 in]
      }
      event "保存按钮": Value Change {
        w275 = u16 1 items=["HPRI"=1, "LPRI"=0] ("priority")
        n103 = event-data() -> ()  [unwired: 1 in, 6 out]
        n104 = call "Enqueue Element Array.vi"("priority"=w275, "queue index"=0, "error in"=w272, "master data"="程序参数保存", "queue in"=w273) -> ("error out"=w270:errorcluster, "queue out"=w271:T11)  [unwired: 5 in]
      }
      event "获取图像": Value Change {
        w283 = u16 1 items=["HPRI"=1, "LPRI"=0] ("priority")
        n105 = event-data() -> ()  [unwired: 1 in, 6 out]
        n106 = property on="Main" class="TabCtl (严格)"("Value"=enum32{"主参数", "模板匹配参数 ", "CCD2 ROI参数", "测试效果"}."测试效果" ("Main")) -> ()  [unwired: 2 in, 2 out]
        n107 = call "Enqueue Element Array.vi"("priority"=w283, "queue index"=0, "error in"=w280, "master data"="获取图像", "queue in"=w281) -> ("error out"=w278:errorcluster, "queue out"=w279:T11)  [unwired: 5 in]
      }
      event "保存图像": Value Change {
        w290 = u16 1 items=["HPRI"=1, "LPRI"=0] ("priority")
        n108 = event-data() -> ()  [unwired: 1 in, 6 out]
        n109 = call "Enqueue Element Array.vi"("priority"=w290, "queue index"=0, "error in"=w287, "master data"="保存图像", "queue in"=w288) -> ("error out"=w285:errorcluster, "queue out"=w286:T11)  [unwired: 5 in]
      }
      event "创建模板": Value Change {
        w297 = u16 1 items=["HPRI"=1, "LPRI"=0] ("priority")
        n110 = event-data() -> ()  [unwired: 1 in, 6 out]
        n111 = call "Enqueue Element Array.vi"("priority"=w297, "queue index"=0, "error in"=w294, "master data"="创建模板", "queue in"=w295) -> ("error out"=w292:errorcluster, "queue out"=w293:T11)  [unwired: 5 in]
      }
      event "ROI LINE 获取": Value Change {
        w305 = u16 1 items=["HPRI"=1, "LPRI"=0] ("priority")
        n112 = event-data() -> ()  [unwired: 1 in, 6 out]
        n113 = property on="Main" class="TabCtl (严格)"("Value"=enum32{"主参数", "模板匹配参数 ", "CCD2 ROI参数", "测试效果"}."测试效果" ("Main")) -> ()  [unwired: 2 in, 2 out]
        n114 = call "Enqueue Element Array.vi"("priority"=w305, "queue index"=0, "error in"=w302, "master data"="ROI LINE 获取", "queue in"=w303) -> ("error out"=w300:errorcluster, "queue out"=w301:T11)  [unwired: 5 in]
      }
      event "ROI BIG 获取": Value Change {
        w313 = u16 1 items=["HPRI"=1, "LPRI"=0] ("priority")
        n115 = event-data() -> ()  [unwired: 1 in, 6 out]
        n116 = property on="Main" class="TabCtl (严格)"("Value"=enum32{"主参数", "模板匹配参数 ", "CCD2 ROI参数", "测试效果"}."测试效果" ("Main")) -> ()  [unwired: 2 in, 2 out]
        n117 = call "Enqueue Element Array.vi"("priority"=w313, "queue index"=0, "error in"=w310, "master data"="ROI BIG 获取", "queue in"=w311) -> ("error out"=w308:errorcluster, "queue out"=w309:T11)  [unwired: 5 in]
      }
      event "测试按钮": Value Change {
        w321 = u16 1 items=["HPRI"=1, "LPRI"=0] ("priority")
        n118 = event-data() -> ()  [unwired: 1 in, 6 out]
        n119 = property on="Main" class="TabCtl (严格)"("Value"=enum32{"主参数", "模板匹配参数 ", "CCD2 ROI参数", "测试效果"}."测试效果" ("Main")) -> ()  [unwired: 2 in, 2 out]
        n120 = call "Enqueue Element Array.vi"("priority"=w321, "queue index"=0, "error in"=w318, "master data"="测试按钮", "queue in"=w319) -> ("error out"=w316:errorcluster, "queue out"=w317:T11)  [unwired: 5 in]
      }
      event "刷新": Value Change {
        w324 = u16 1 items=["HPRI"=1, "LPRI"=0] ("priority")
        n121 = event-data() -> ()  [unwired: 1 in, 6 out]
        n122 = property on="Main" class="TabCtl (严格)"("Value"=enum32{"主参数", "模板匹配参数 ", "CCD2 ROI参数", "测试效果"}."模板匹配参数 " ("Main")) -> ()  [unwired: 2 in, 2 out]
        n123 = call "Enqueue Element Array.vi"("priority"=w324, "queue index"=0, "error in"=w329, "master data"="刷新", "queue in"=w330) -> ("error out"=w327:errorcluster, "queue out"=w328:T11)  [unwired: 5 in]
      }
    }
    n124 = call "GetSystemTime.vi"() -> ("date/time string"=→"system time":string)  [unwired: 7 in]
  }
  n125 = call "Release Queue Array.vi"("error in"=w3, "queue in"=w1) -> ("error out"=w2:errorcluster)  [unwired: 2 in, 3 out]
  n126 = call "Release Queue Array.vi"("error in"=w6, "queue in"=w1) -> ("error out"=w9:errorcluster)  [unwired: 2 in, 3 out]
  n127 = call "MergeErrors.vi"("error in 3 (no error)"=w2, "error in 4 (no error)"=w9) -> ("error out"=w8:errorcluster)  [unwired: 6 in]
  n128 = call "ExitAppMode.vi"("error in (no error)"=w8) -> ("error out"=w7:errorcluster)  [unwired: 10 in]
  n129 = call <vilib>:"Clear Errors.vi"("error in (no error)"=w7) -> ()  [unwired: 5 in, 2 out]
